vi "TestAllWritings.vi"() -> ()   [LabVIEW 2017]
uses:
  InputRange.ctl
  InputType.ctl
  InputMode.ctl
  InputCouple.ctl
  InputFilter.ctl
  InputGround.ctl
  InputSensitivity.ctl
  InputTimeConstant.ctl
  OutputChannelSignal.ctl
  OutputChannel.ctl
  OutSineReference.ctl
  OutSineSource.ctl
panel:
  out "OutSineSource":T1 caption="Out sine ref" items=["Internal", "External", "Dual", "Chop"]
  out "OutSineRef":T2 caption="Out sine ref" items=["Common", "Difference"]
  out "Offset":dbl caption="Offset, V"
  out "Frequency":dbl caption="Frequency, Hz"
  out "Amplitude":dbl caption="Amplitude, V"
  in  "OutputChannel":T3 caption="Output channel" items=["Channel 1", "Channel 2"]
  out "OutputChannelSignal":T4 caption="Output channel signal" items=["X (ch1) / Y (ch2)", "R (ch1) / Q (ch2)"]
  out "InputTimeConstant":T5=2 caption="Input time constant" items=["1 us", "3 us", "10 us", "30 us", "100 us", "300 us", "1 ms", "3 ms", "10 ms", "30 ms", "100 ms", "300 ms", "1 s", "3 s", "10 s", "30 s", "100 s", "300 s", "1 Ks", "3 Ks", "10 Ks", "30 Ks"]
  out "InputSensitivity":T6=26 caption="Input sensitivity" items=["1 V [uA]", "500 mV [nA]", "200 mV [nA]", "100 mV [nA]", "50 mV [nA]", "20 mV [nA]", "10 mV [nA]", "5 mV [nA]", "2 mV [nA]", "1 mV [nA]", "500 uV [pA]", "200 uV [pA]", "100 uV [pA]", "50 uV [pA]", "20 uV [pA]", "10 uV [pA]", "5 uV [pA]", "2 uV [pA]", "1 uV [pA]", "500 nV [fA]", "200 nV [fA]", "100 nV [fA]", "50 nV [fA]", "20 nV [fA]", "10 nV [fA]", "5 nV [fA]", "2 nV [fA]", "1 nV [fA]"]
  out "InputGround":T7 caption="Input ground" items=["Float", "Ground"]
  out "InputFilter":T8 caption="Input filter" items=["6 db/oct", "12 db/oct", "18 db/oct", "24 db/oct"]
  out "InputCouple":T9 caption="Input couple" items=["AC", "DC"]
  out "InputMode":T10 caption="Input mode" items=["A", "A-B"]
  out "InputType":T11=2 caption="Input type" items=["Voltage", "Current"]
  out "InputRange":T12=2 caption="Input range" items=["1 V", "300 mV", "100 mV", "30 mV", "10 mV"]
  in  "VISA resource name":refnum<visa-resource-name>
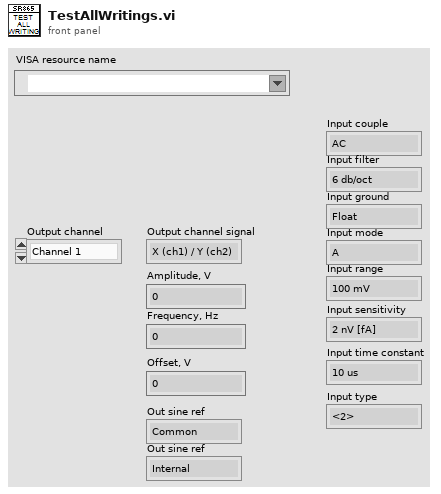
[diagram p1: front panel]
types:
  T1 = typedef "OutSineSource.ctl" = u16
  T2 = typedef "OutSineReference.ctl" = u16
  T3 = typedef "OutputChannel.ctl" = u16
  T4 = typedef "OutputChannelSignal.ctl" = u16
  T5 = typedef "InputTimeConstant.ctl" = u16
  T6 = typedef "InputSensitivity.ctl" = u16
  T7 = typedef "InputGround.ctl" = u16
  T8 = typedef "InputFilter.ctl" = u16
  T9 = typedef "InputCouple.ctl" = u16
  T10 = typedef "InputMode.ctl" = u16
  T11 = typedef "InputType.ctl" = u16
  T12 = typedef "InputRange.ctl" = u16
  T13 = typedef "SR865.ctl" = cluster{"VISA resource name":refnum<visa-resource-name>, "ReadWrite":T14}
  T14 = typedef "Semaphore RefNum" = refnum<k1>
  T15 = typedef "LVStringsAndValuesArrayTypeDef_U16.ctl" = cluster{"String":string, "Value":u16}[]
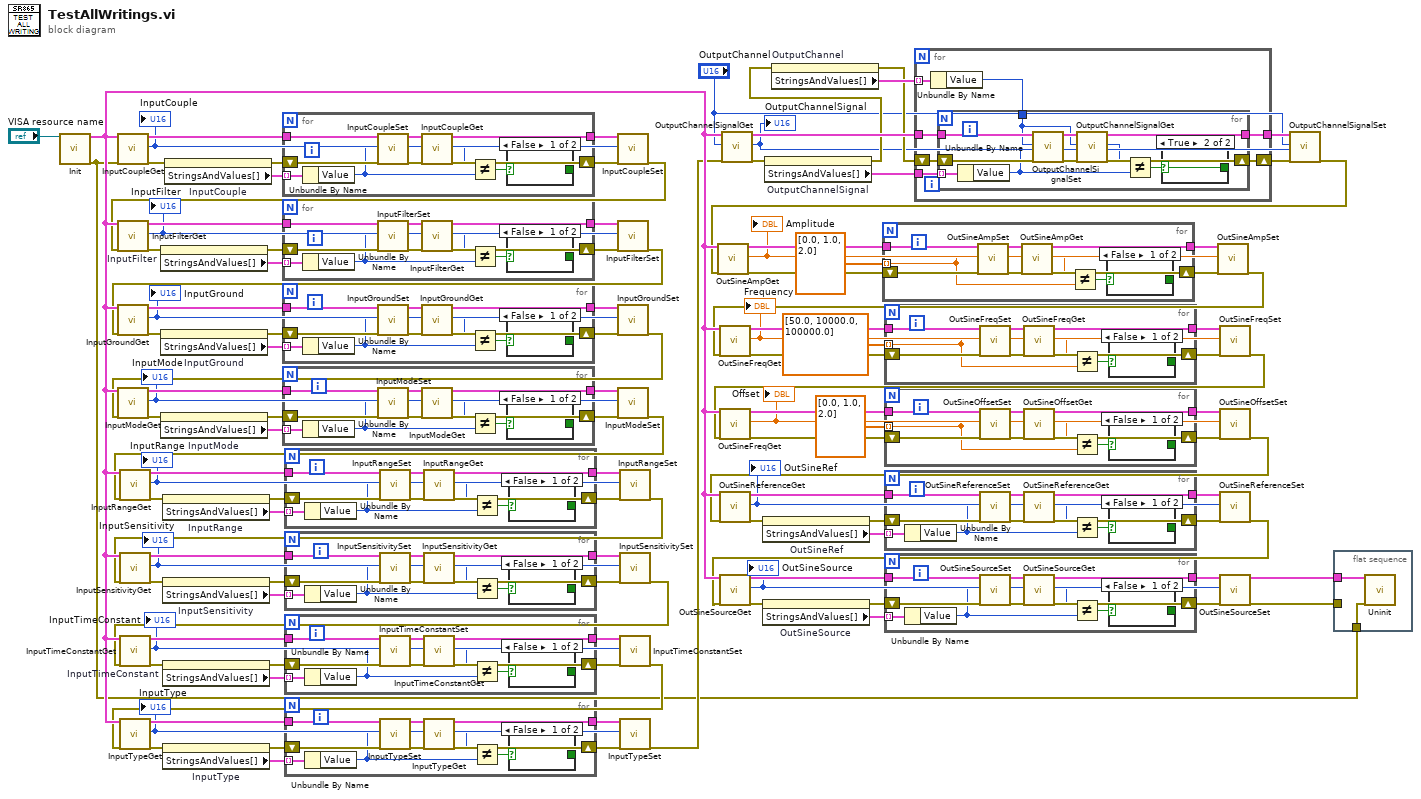
[diagram p0: block diagram]
diagram:
  n1 = call "Init.vi"("VISA resource name"="VISA resource name") -> ("SR865"=w33:T13, "error out"=w1:errorcluster)  [unwired: 17 in]
  n2 = call "InputCoupleGet.vi"("SR865 in"=w33, "error in"=w1) -> ("SR865 out"=w114:T13, "InputCouple"=w109:T9, "error out"=w115:errorcluster)  [unwired: 15 in]
  "InputCouple" <- w109
  n3 = property on="InputCouple" class="Ring (strict)"(error in=w115) -> (error out=w112:errorcluster, "StringsAndValues[]"=w113:T15)  [unwired: 1 in, 1 out]
  n4 = for {
    tunnel: w113 -> [w126] mode=indexing
    tunnel: w114 -> [w125]
    tunnel: [w121] -> w110
    shift-right: [w120] -> w111
    shift-left: w112 -> [w124]
    n5 = Unbundle By Name(w126) -> ("Value"=w118:u16)
    n6 = call "InputCoupleSet.vi"("SR865 in"=w125, "InputCouple"=w118, "error in"=w124) -> ("SR865 out"=w123:T13, "error out"=w122:errorcluster)  [unwired: 15 in]
    n7 = call "InputCoupleGet.vi"("SR865 in"=w123, "error in"=w122) -> ("SR865 out"=w121:T13, "InputCouple"=w119:T9, "error out"=w120:errorcluster)  [unwired: 15 in]
    n8 = Not Equal?(x=w119, y=w118) -> (x != y?=w117:bool)
    n9 = case shown="False" w117 {
      selector: w117 -> [_ w127]
      tunnel: [_ w127] -> _
      frame False {
      }
      frame True {
      }
    }
  }
  n10 = call "InputCoupleSet.vi"("SR865 in"=w110, "InputCouple"=w109, "error in"=w111) -> ("error out"=w16:errorcluster)  [unwired: 15 in, 1 out]
  n11 = call "InputFilterGet.vi"("SR865 in"=w33, "error in"=w16) -> ("SR865 out"=w108:T13, "InputFilter"=w105:T8, "error out"=w104:errorcluster)  [unwired: 15 in]
  "InputFilter" <- w105
  n12 = property on="InputFilter" class="Ring (strict)"(error in=w104) -> (error out=w102:errorcluster, "StringsAndValues[]"=w103:T15)  [unwired: 1 in, 1 out]
  n13 = for {
    tunnel: w103 -> [w137] mode=indexing
    tunnel: w108 -> [w136]
    tunnel: [w132] -> w106
    shift-right: [w131] -> w107
    shift-left: w102 -> [w135]
    n14 = Unbundle By Name(w137) -> ("Value"=w129:u16)
    n15 = call "InputFilterSet.vi"("SR865 in"=w136, "InputFilter"=w129, "error in"=w135) -> ("SR865 out"=w134:T13, "error out"=w133:errorcluster)  [unwired: 15 in]
    n16 = call "InputFilterGet.vi"("SR865 in"=w134, "error in"=w133) -> ("SR865 out"=w132:T13, "InputFilter"=w130:T8, "error out"=w131:errorcluster)  [unwired: 15 in]
    n17 = Not Equal?(x=w130, y=w129) -> (x != y?=w128:bool)
    n18 = case shown="False" w128 {
      selector: w128 -> [_ w138]
      tunnel: [_ w138] -> _
      frame False {
      }
      frame True {
      }
    }
  }
  n19 = call "InputFilterSet.vi"("SR865 in"=w106, "InputFilter"=w105, "error in"=w107) -> ("error out"=w15:errorcluster)  [unwired: 15 in, 1 out]
  n20 = call "InputGroundGet.vi"("SR865 in"=w33, "error in"=w15) -> ("SR865 out"=w101:T13, "InputGround"=w95:T7, "error out"=w98:errorcluster)  [unwired: 15 in]
  "InputGround" <- w95
  n21 = property on="InputGround" class="Ring (strict)"(error in=w98) -> (error out=w96:errorcluster, "StringsAndValues[]"=w97:T15)  [unwired: 1 in, 1 out]
  n22 = for {
    tunnel: w97 -> [w148] mode=indexing
    tunnel: w101 -> [w147]
    tunnel: [w143] -> w99
    shift-right: [w142] -> w100
    shift-left: w96 -> [w146]
    n23 = Unbundle By Name(w148) -> ("Value"=w140:u16)
    n24 = call "InputGroundSet.vi"("SR865 in"=w147, "InputGround"=w140, "error in"=w146) -> ("SR865 out"=w145:T13, "error out"=w144:errorcluster)  [unwired: 15 in]
    n25 = call "InputGroundGet.vi"("SR865 in"=w145, "error in"=w144) -> ("SR865 out"=w143:T13, "InputGround"=w141:T7, "error out"=w142:errorcluster)  [unwired: 15 in]
    n26 = Not Equal?(x=w141, y=w140) -> (x != y?=w139:bool)
    n27 = case shown="False" w139 {
      selector: w139 -> [_ w149]
      tunnel: [_ w149] -> _
      frame False {
      }
      frame True {
      }
    }
  }
  n28 = call "InputGroundSet.vi"("SR865 in"=w99, "InputGround"=w95, "error in"=w100) -> ("error out"=w14:errorcluster)  [unwired: 15 in, 1 out]
  n29 = call "InputModeGet.vi"("SR865 in"=w33, "error in"=w14) -> ("SR865 out"=w94:T13, "InputMode"=w64:T10, "error out"=w91:errorcluster)  [unwired: 15 in]
  "InputMode" <- w64
  n30 = property on="InputMode" class="Ring (strict)"(error in=w91) -> (error out=w89:errorcluster, "StringsAndValues[]"=w90:T15)  [unwired: 1 in, 1 out]
  n31 = for {
    tunnel: w90 -> [w159] mode=indexing
    tunnel: w94 -> [w158]
    tunnel: [w154] -> w92
    shift-right: [w153] -> w93
    shift-left: w89 -> [w157]
    n32 = Unbundle By Name(w159) -> ("Value"=w151:u16)
    n33 = call "InputModeSet.vi"("SR865 in"=w158, "InputMode"=w151, "error in"=w157) -> ("SR865 out"=w156:T13, "error out"=w155:errorcluster)  [unwired: 15 in]
    n34 = call "InputModeGet.vi"("SR865 in"=w156, "error in"=w155) -> ("SR865 out"=w154:T13, "InputMode"=w152:T10, "error out"=w153:errorcluster)  [unwired: 15 in]
    n35 = Not Equal?(x=w152, y=w151) -> (x != y?=w150:bool)
    n36 = case shown="False" w150 {
      selector: w150 -> [_ w160]
      tunnel: [_ w160] -> _
      frame False {
      }
      frame True {
      }
    }
  }
  n37 = call "InputModeSet.vi"("SR865 in"=w92, "InputMode"=w64, "error in"=w93) -> ("error out"=w13:errorcluster)  [unwired: 15 in, 1 out]
  n38 = call "InputRangeGet.vi"("SR865 in"=w33, "error in"=w13) -> ("SR865 out"=w88:T13, "InputRange"=w63:T12, "error out"=w85:errorcluster)  [unwired: 15 in]
  "InputRange" <- w63
  n39 = property on="InputRange" class="Ring (strict)"(error in=w85) -> (error out=w83:errorcluster, "StringsAndValues[]"=w84:T15)  [unwired: 1 in, 1 out]
  n40 = for {
    tunnel: w84 -> [w170] mode=indexing
    tunnel: w88 -> [w169]
    tunnel: [w165] -> w86
    shift-right: [w164] -> w87
    shift-left: w83 -> [w168]
    n41 = Unbundle By Name(w170) -> ("Value"=w162:u16)
    n42 = call "InputRangeSet.vi"("SR865 in"=w169, "InputRange"=w162, "error in"=w168) -> ("SR865 out"=w167:T13, "error out"=w166:errorcluster)  [unwired: 15 in]
    n43 = call "InputRangeGet.vi"("SR865 in"=w167, "error in"=w166) -> ("SR865 out"=w165:T13, "InputRange"=w163:T12, "error out"=w164:errorcluster)  [unwired: 15 in]
    n44 = Not Equal?(x=w163, y=w162) -> (x != y?=w161:bool)
    n45 = case shown="False" w161 {
      selector: w161 -> [_ w171]
      tunnel: [_ w171] -> _
      frame False {
      }
      frame True {
      }
    }
  }
  n46 = call "InputRangeSet.vi"("SR865 in"=w86, "InputRange"=w63, "error in"=w87) -> ("error out"=w12:errorcluster)  [unwired: 15 in, 1 out]
  n47 = call "InputSensitivityGet.vi"("SR865 in"=w33, "error in"=w12) -> ("SR865 out"=w82:T13, "InputSensitivity"=w62:T6, "error out"=w79:errorcluster)  [unwired: 15 in]
  "InputSensitivity" <- w62
  n48 = property on="InputSensitivity" class="Ring (strict)"(error in=w79) -> (error out=w77:errorcluster, "StringsAndValues[]"=w78:T15)  [unwired: 1 in, 1 out]
  n49 = for {
    tunnel: w78 -> [w181] mode=indexing
    tunnel: w82 -> [w180]
    tunnel: [w176] -> w80
    shift-right: [w175] -> w81
    shift-left: w77 -> [w179]
    n50 = Unbundle By Name(w181) -> ("Value"=w173:u16)
    n51 = call "InputSensitivitySet.vi"("SR865 in"=w180, "InputSensitivity"=w173, "error in"=w179) -> ("SR865 out"=w178:T13, "error out"=w177:errorcluster)  [unwired: 15 in]
    n52 = call "InputSensitivityGet.vi"("SR865 in"=w178, "error in"=w177) -> ("SR865 out"=w176:T13, "InputSensitivity"=w174:T6, "error out"=w175:errorcluster)  [unwired: 15 in]
    n53 = Not Equal?(x=w174, y=w173) -> (x != y?=w172:bool)
    n54 = case shown="False" w172 {
      selector: w172 -> [_ w182]
      tunnel: [_ w182] -> _
      frame False {
      }
      frame True {
      }
    }
  }
  n55 = call "InputSensitivitySet.vi"("SR865 in"=w80, "InputSensitivity"=w62, "error in"=w81) -> ("error out"=w11:errorcluster)  [unwired: 15 in, 1 out]
  n56 = call "InputTimeConstantGet.vi"("SR865 in"=w33, "error in"=w11) -> ("SR865 out"=w76:T13, "InputTimeConstant"=w61:T5, "error out"=w73:errorcluster)  [unwired: 15 in]
  "InputTimeConstant" <- w61
  n57 = property on="InputTimeConstant" class="Ring (strict)"(error in=w73) -> (error out=w71:errorcluster, "StringsAndValues[]"=w72:T15)  [unwired: 1 in, 1 out]
  n58 = for {
    tunnel: w72 -> [w192] mode=indexing
    tunnel: w76 -> [w191]
    tunnel: [w187] -> w74
    shift-right: [w186] -> w75
    shift-left: w71 -> [w190]
    n59 = Unbundle By Name(w192) -> ("Value"=w184:u16)
    n60 = call "InputTimeConstantSet.vi"("SR865 in"=w191, "InputTimeConstant"=w184, "error in"=w190) -> ("SR865 out"=w189:T13, "error out"=w188:errorcluster)  [unwired: 15 in]
    n61 = call "InputTimeConstantGet.vi"("SR865 in"=w189, "error in"=w188) -> ("SR865 out"=w187:T13, "InputTimeConstant"=w185:T5, "error out"=w186:errorcluster)  [unwired: 15 in]
    n62 = Not Equal?(x=w185, y=w184) -> (x != y?=w183:bool)
    n63 = case shown="False" w183 {
      selector: w183 -> [_ w193]
      tunnel: [_ w193] -> _
      frame False {
      }
      frame True {
      }
    }
  }
  n64 = call "InputTimeConstantSet.vi"("SR865 in"=w74, "InputTimeConstant"=w61, "error in"=w75) -> ("error out"=w10:errorcluster)  [unwired: 15 in, 1 out]
  n65 = call "InputTypeGet.vi"("SR865 in"=w33, "error in"=w10) -> ("SR865 out"=w70:T13, "InputType"=w60:T11, "error out"=w67:errorcluster)  [unwired: 15 in]
  "InputType" <- w60
  n66 = property on="InputType" class="Ring (strict)"(error in=w67) -> (error out=w65:errorcluster, "StringsAndValues[]"=w66:T15)  [unwired: 1 in, 1 out]
  n67 = for {
    tunnel: w66 -> [w203] mode=indexing
    tunnel: w70 -> [w202]
    tunnel: [w198] -> w68
    shift-right: [w197] -> w69
    shift-left: w65 -> [w201]
    n68 = Unbundle By Name(w203) -> ("Value"=w195:u16)
    n69 = call "InputTypeSet.vi"("SR865 in"=w202, "InputType"=w195, "error in"=w201) -> ("SR865 out"=w200:T13, "error out"=w199:errorcluster)  [unwired: 15 in]
    n70 = call "InputTypeGet.vi"("SR865 in"=w200, "error in"=w199) -> ("SR865 out"=w198:T13, "InputType"=w196:T11, "error out"=w197:errorcluster)  [unwired: 15 in]
    n71 = Not Equal?(x=w196, y=w195) -> (x != y?=w194:bool)
    n72 = case shown="False" w194 {
      selector: w194 -> [_ w204]
      tunnel: [_ w204] -> _
      frame False {
      }
      frame True {
      }
    }
  }
  n73 = call "InputTypeSet.vi"("SR865 in"=w68, "InputType"=w60, "error in"=w69) -> ("error out"=w9:errorcluster)  [unwired: 15 in, 1 out]
  n74 = call "OutputChannelSignalGet.vi"("SR865 in"=w33, "OutputChannel"="OutputChannel", "error in"=w9) -> ("SR865 out"=w59:T13, "OutputChannelSignal"=w28:T4, "error out"=w56:errorcluster)  [unwired: 14 in]
  "OutputChannelSignal" <- w28
  n75 = property on="OutputChannelSignal" class="Ring (strict)"(error in=w56) -> (error out=w31:errorcluster, "StringsAndValues[]"=w55:T15)  [unwired: 1 in, 1 out]
  n76 = property on="OutputChannel" class="Ring (strict)"(error in=w31) -> (error out=w30:errorcluster, "StringsAndValues[]"=w32:T15)  [unwired: 1 in, 1 out]
  n77 = for {
    tunnel: w59 -> [w211]
    tunnel: [w209] -> w57
    tunnel: w55 -> [w208]
    shift-right: [w210] -> w58
    shift-left: w30 -> [w207]
    tunnel: w32 -> [w206] mode=indexing
    n78 = Unbundle By Name(w206) -> ("Value"=w205:u16)
    n79 = for {
      tunnel: w208 -> [w222] mode=indexing
      tunnel: w211 -> [w221]
      tunnel: [w217] -> w209
      shift-right: [w216] -> w210
      shift-left: w207 -> [w220]
      tunnel: w205 -> [w212]
      n80 = Unbundle By Name(w222) -> ("Value"=w213:u16)
      n81 = call "OutputChannelSignalSet.vi"("SR865 in"=w221, "OutputChannel"=w212, "OutputChannelSignal"=w213, "error in"=w220) -> ("SR865 out"=w219:T13, "error out"=w218:errorcluster)  [unwired: 14 in]
      n82 = call "OutputChannelSignalGet.vi"("SR865 in"=w219, "OutputChannel"=w212, "error in"=w218) -> ("SR865 out"=w217:T13, "OutputChannelSignal"=w215:T4, "error out"=w216:errorcluster)  [unwired: 14 in]
      n83 = Not Equal?(x=w215, y=w213) -> (x != y?=w214:bool)
      n84 = case shown="True" w214 {
        selector: w214 -> [_ w223]
        tunnel: [_ w223] -> _
        frame False {
        }
        frame True {
        }
      }
    }
  }
  n85 = call "OutputChannelSignalSet.vi"("SR865 in"=w57, "OutputChannel"="OutputChannel", "OutputChannelSignal"=w28, "error in"=w58) -> ("error out"=w8:errorcluster)  [unwired: 14 in, 1 out]
  n86 = call "OutSineAmpGet.vi"("SR865 in"=w33, "error in"=w8) -> ("SR865 out"=w54:T13, "Amplitude"=w26:dbl, "error out"=w27:errorcluster)  [unwired: 15 in]
  "Amplitude" <- w26
  n87 = for {
    tunnel: w54 -> [w232]
    tunnel: [w228] -> w52
    shift-right: [w227] -> w53
    shift-left: w27 -> [w231]
    tunnel: dbl[] [0.0, 1.0, 2.0] -> [w224] mode=indexing
    n88 = call "OutSineAmpSet.vi"("SR865 in"=w232, "Amplitude"=w224, "error in"=w231) -> ("SR865 out"=w230:T13, "error out"=w229:errorcluster)  [unwired: 15 in]
    n89 = call "OutSineAmpGet.vi"("SR865 in"=w230, "error in"=w229) -> ("SR865 out"=w228:T13, "Amplitude"=w226:dbl, "error out"=w227:errorcluster)  [unwired: 15 in]
    n90 = Not Equal?(x=w226, y=w224) -> (x != y?=w225:bool)
    n91 = case shown="False" w225 {
      selector: w225 -> [_ w233]
      tunnel: [_ w233] -> _
      frame False {
      }
      frame True {
      }
    }
  }
  n92 = call "OutSineAmpSet.vi"("SR865 in"=w52, "Amplitude"=w26, "error in"=w53) -> ("error out"=w7:errorcluster)  [unwired: 15 in, 1 out]
  n93 = call "OutSineFreqGet.vi"("SR865 in"=w33, "error in"=w7) -> ("SR865 out"=w51:T13, "Frequency"=w24:dbl, "error out"=w22:errorcluster)  [unwired: 15 in]
  "Frequency" <- w24
  n94 = for {
    tunnel: w51 -> [w242]
    tunnel: [w238] -> w49
    shift-right: [w237] -> w50
    shift-left: w22 -> [w241]
    tunnel: dbl[] [50.0, 10000.0, 100000.0] -> [w234] mode=indexing
    n95 = call "OutSineFreqSet.vi"("SR865 in"=w242, "Frequency"=w234, "error in"=w241) -> ("SR865 out"=w240:T13, "error out"=w239:errorcluster)  [unwired: 15 in]
    n96 = call "OutSineFreqGet.vi"("SR865 in"=w240, "error in"=w239) -> ("SR865 out"=w238:T13, "Frequency"=w236:dbl, "error out"=w237:errorcluster)  [unwired: 15 in]
    n97 = Not Equal?(x=w236, y=w234) -> (x != y?=w235:bool)
    n98 = case shown="False" w235 {
      selector: w235 -> [_ w243]
      tunnel: [_ w243] -> _
      frame False {
      }
      frame True {
      }
    }
  }
  n99 = call "OutSineFreqSet.vi"("SR865 in"=w49, "Frequency"=w24, "error in"=w50) -> ("error out"=w6:errorcluster)  [unwired: 15 in, 1 out]
  n100 = call "OutSineFreqGet.vi"("SR865 in"=w33, "error in"=w6) -> ("SR865 out"=w48:T13, "Frequency"=w21:dbl, "error out"=w5:errorcluster)  [unwired: 15 in]
  "Offset" <- w21
  n101 = for {
    tunnel: w48 -> [w252]
    tunnel: [w248] -> w46
    shift-right: [w247] -> w47
    shift-left: w5 -> [w251]
    tunnel: dbl[] [0.0, 1.0, 2.0] -> [w244] mode=indexing
    n102 = call "OutSineOffsetSet.vi"("SR865 in"=w252, "Amplitude"=w244, "error in"=w251) -> ("SR865 out"=w250:T13, "error out"=w249:errorcluster)  [unwired: 15 in]
    n103 = call "OutSineOffsetGet.vi"("SR865 in"=w250, "error in"=w249) -> ("SR865 out"=w248:T13, "Offset"=w246:dbl, "error out"=w247:errorcluster)  [unwired: 15 in]
    n104 = Not Equal?(x=w246, y=w244) -> (x != y?=w245:bool)
    n105 = case shown="False" w245 {
      selector: w245 -> [_ w253]
      tunnel: [_ w253] -> _
      frame False {
      }
      frame True {
      }
    }
  }
  n106 = call "OutSineOffsetSet.vi"("SR865 in"=w46, "Amplitude"=w21, "error in"=w47) -> ("error out"=w4:errorcluster)  [unwired: 15 in, 1 out]
  n107 = call "OutSineReferenceGet.vi"("SR865 in"=w33, "error in"=w4) -> ("SR865 out"=w45:T13, "OutSineRef"=w19:T2, "error out"=w42:errorcluster)  [unwired: 15 in]
  "OutSineRef" <- w19
  n108 = property on="OutSineRef" class="Ring (strict)"(error in=w42) -> (error out=w40:errorcluster, "StringsAndValues[]"=w41:T15)  [unwired: 1 in, 1 out]
  n109 = for {
    tunnel: w41 -> [w263] mode=indexing
    tunnel: w45 -> [w262]
    tunnel: [w258] -> w43
    shift-right: [w257] -> w44
    shift-left: w40 -> [w261]
    n110 = Unbundle By Name(w263) -> ("Value"=w255:u16)
    n111 = call "OutSineReferenceSet.vi"("SR865 in"=w262, "OutSineRef"=w255, "error in"=w261) -> ("SR865 out"=w260:T13, "error out"=w259:errorcluster)  [unwired: 15 in]
    n112 = call "OutSineReferenceGet.vi"("SR865 in"=w260, "error in"=w259) -> ("SR865 out"=w258:T13, "OutSineRef"=w256:T2, "error out"=w257:errorcluster)  [unwired: 15 in]
    n113 = Not Equal?(x=w256, y=w255) -> (x != y?=w254:bool)
    n114 = case shown="False" w254 {
      selector: w254 -> [_ w264]
      tunnel: [_ w264] -> _
      frame False {
      }
      frame True {
      }
    }
  }
  n115 = call "OutSineReferenceSet.vi"("SR865 in"=w43, "OutSineRef"=w19, "error in"=w44) -> ("error out"=w3:errorcluster)  [unwired: 15 in, 1 out]
  n116 = call "OutSineSourceGet.vi"("SR865 in"=w33, "error in"=w3) -> ("SR865 out"=w39:T13, "OutSineSource"=w18:T1, "error out"=w36:errorcluster)  [unwired: 15 in]
  "OutSineSource" <- w18
  n117 = property on="OutSineSource" class="Ring (strict)"(error in=w36) -> (error out=w34:errorcluster, "StringsAndValues[]"=w35:T15)  [unwired: 1 in, 1 out]
  n118 = for {
    tunnel: w35 -> [w274] mode=indexing
    tunnel: w39 -> [w273]
    tunnel: [w269] -> w37
    shift-right: [w268] -> w38
    shift-left: w34 -> [w272]
    n119 = Unbundle By Name(w274) -> ("Value"=w266:u16)
    n120 = call "OutSineSourceSet.vi"("SR865 in"=w273, "OutSineSource"=w266, "error in"=w272) -> ("SR865 out"=w271:T13, "error out"=w270:errorcluster)  [unwired: 15 in]
    n121 = call "OutSineSourceGet.vi"("SR865 in"=w271, "error in"=w270) -> ("SR865 out"=w269:T13, "OutSineSource"=w267:T1, "error out"=w268:errorcluster)  [unwired: 15 in]
    n122 = Not Equal?(x=w267, y=w266) -> (x != y?=w265:bool)
    n123 = case shown="False" w265 {
      selector: w265 -> [_ w275]
      tunnel: [_ w275] -> _
      frame False {
      }
      frame True {
      }
    }
  }
  n124 = call "OutSineSourceSet.vi"("SR865 in"=w37, "OutSineSource"=w18, "error in"=w38) -> ("SR865 out"=w17:T13, "error out"=w2:errorcluster)  [unwired: 15 in]
  n125 = flat-sequence {
    tunnel: w17 -> [w277]
    tunnel: w2 -> [_]
    tunnel: w1 -> [w276]
    frame #0 {
      n126 = call "Uninit.vi"("SR865 in"=w277, "error in"=w276) -> ()  [unwired: 17 in, 1 out]
    }
  }
